vi "Separador.vi"(7 "Lectura del puerto Serial":string) -> (0 "Propano":dbl, 1 "ALcohol":dbl, 2 "CO":dbl, 3 "LPG":dbl, 4 "H2":dbl, 5 "Humedad":dbl, 6 "Temperatura":dbl)   [LabVIEW 2020]
panel:
  out "Arreglo de Valores":string[](array[string])
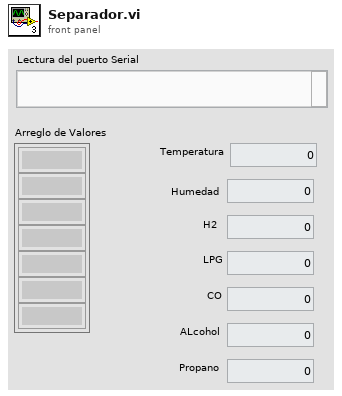
[diagram p1: front panel]
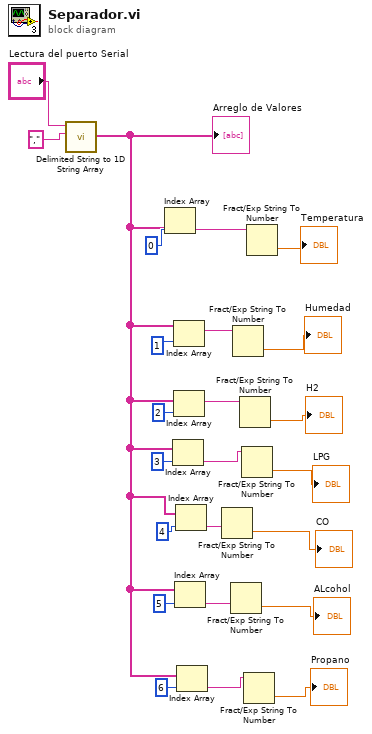
[diagram p0: block diagram]
diagram:
  n1 = call <vilib>:"Delimited String to 1D String Array.vi"("delimiter"="," ("search string/char (-)"), "delimited string"="Lectura del puerto Serial") -> ("string array"=w17:string[])  [unwired: 9 in]
  "Arreglo de Valores" <- w17
  n2 = Index Array(array=w17, index=0) -> (element=w22:string)
  n3 = Index Array(array=w17, index=3) -> (element=w10:string)
  n4 = Index Array(array=w17, index=1) -> (element=w19:string)
  n5 = Index Array(array=w17, index=2) -> (element=w11:string)
  n6 = Index Array(array=w17, index=5) -> (element=w8:string)
  n7 = Index Array(array=w17, index=4) -> (element=w9:string)
  n8 = Index Array(array=w17, index=6) -> (element=w7:string)
  n9 = Fract/Exp String To Number(string=w9) -> (number=→"CO":dbl)  [unwired: 3 in, 1 out]
  n10 = Fract/Exp String To Number(string=w8) -> (number=→"ALcohol":dbl)  [unwired: 3 in, 1 out]
  n11 = Fract/Exp String To Number(string=w19) -> (number=→"Humedad":dbl)  [unwired: 3 in, 1 out]
  n12 = Fract/Exp String To Number(string=w11) -> (number=→"H2":dbl)  [unwired: 3 in, 1 out]
  n13 = Fract/Exp String To Number(string=w10) -> (number=→"LPG":dbl)  [unwired: 3 in, 1 out]
  n14 = Fract/Exp String To Number(string=w7) -> (number=→"Propano":dbl)  [unwired: 3 in, 1 out]
  n15 = Fract/Exp String To Number(string=w22) -> (number=→"Temperatura":dbl)  [unwired: 3 in, 1 out]
